vi "test Scripted Hardware Configuration.vi"(8 "error in (no error)":errorcluster, 11 "TestCase in":refnum<class "Hardware Configuration.lvclass">) -> (0 "error out":errorcluster, 3 "TestCase out":refnum<class "Hardware Configuration.lvclass">)   [LabVIEW 2020, in "Hardware Configuration.lvclass"]
uses:
  Hardware Configuration.lvclass
  <vilib>/addons/_JKI Toolkits/VI Tester/TestCase.llb/TestCase.lvclass
  niveristand-custom-device-testing-tools/Source/VeriStandTestUtilities/VeriStandTestUtilities.lvlib
  Scripting/Ballard/Ballard ARINC 429 Scripting.lvlib
  Hardware Configuration/Ballard ARINC 429 Hardware Configuration.lvlib
  C:/Program Files (x86)/National Instruments/LabVIEW 2020/vi.lib/addons/_JKI Toolkits/VI Tester/TestCase.llb/TestCase.lvclass
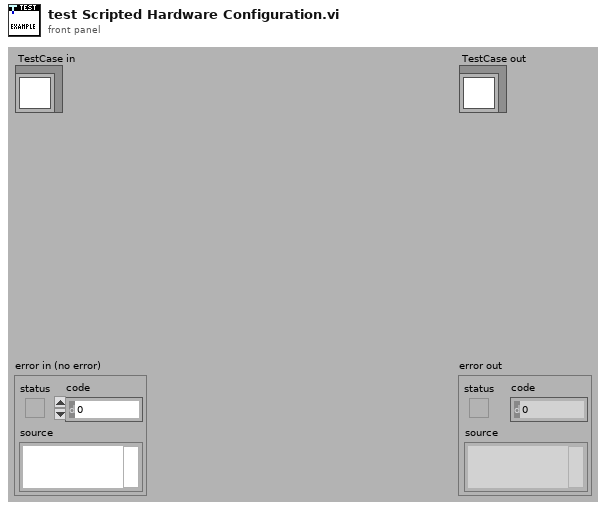
[diagram p1: front panel]
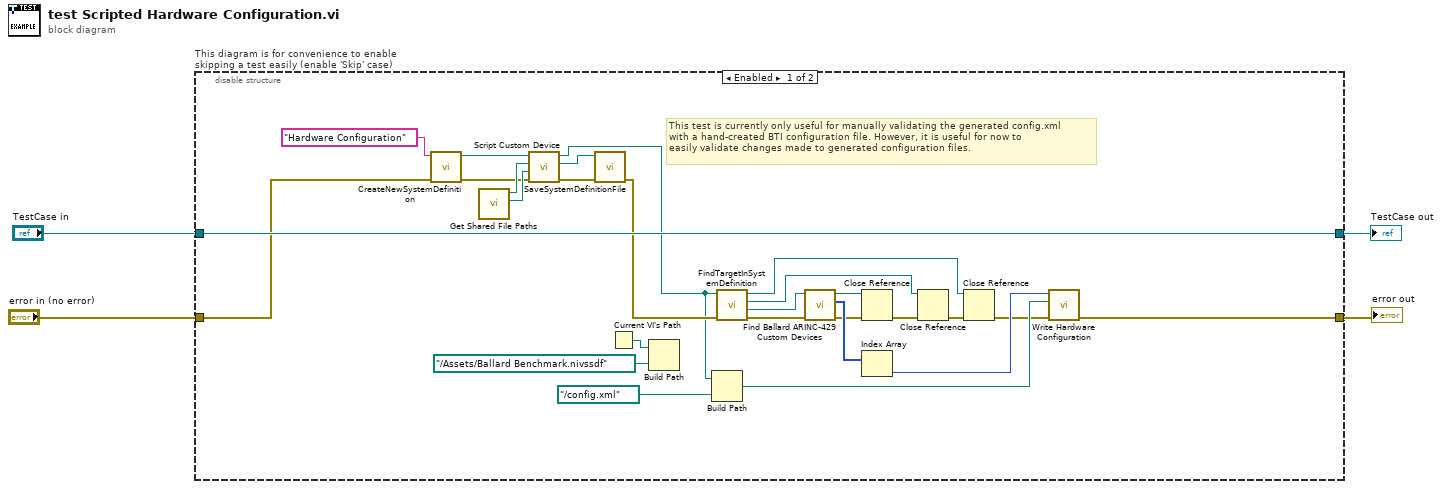
[diagram p0: block diagram]
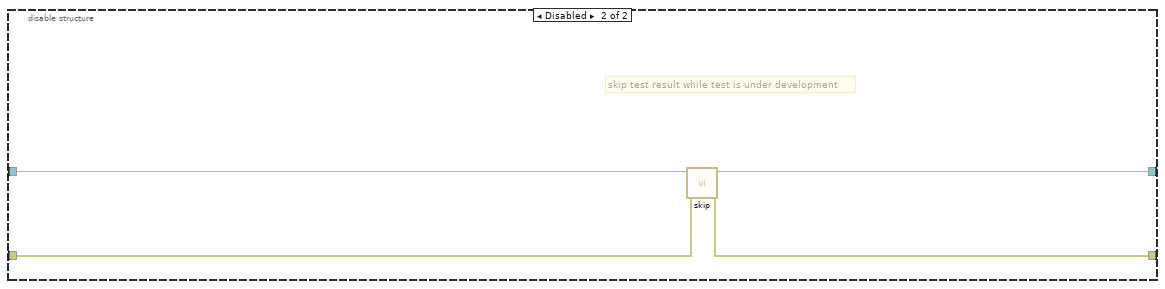
[diagram p2: hidden frame]
diagram:
  n1 = disable-structure "This diagram is for convenience to enable skipping a test easily (enable 'Skip' case)" shown="Enabled" {
    disable-tunnel: "TestCase in" -> [w31 w35]
    disable-tunnel: [w31 w33] -> w1
    disable-tunnel: [w17 w34] -> w3
    disable-tunnel: "error in (no error)" -> [w7 w32]
    frame Enabled {
      # "This test is currently only useful for manually validating the generated config.xml\nwith a hand-created BTI configuration file. However, it is useful for now to\neasily validate changes made to generated configuration files."
      n2 = call "CreateNewSystemDefinition.vi"("error in"=w7, "System Definition Name"="Hardware Configuration" ("Channel")) -> ("error out"=w10:errorcluster, "System Definition Path"=w12:path)  [unwired: 8 in]
      n3 = call "Get Shared File Paths.vi"() -> ("Hardware File"=w14:path, "Parameters File"=w13:path)  [unwired: 10 in]
      n4 = call "Script Custom Device.vi"("error in"=w10, "Hardware Configuration File Path"=w14, "Parameters Configuration File Path"=w13, "System Definition File Path In"=w12) -> ("error out"=w9:errorcluster, "System Definition Reference"=w11:refnum<k24>, "System Definition File Path Out"=w5:path)  [unwired: 4 in, 1 out]
      n5 = call "SaveSystemDefinitionFile.vi"("error in (no error)"=w9, "System Definition Reference in"=w11) -> ("error out"=w6:errorcluster)  [unwired: 8 in, 1 out]
      n6 = Current VI's Path() -> (path=w30:path)
      n7 = Build Path(base path=w30, name or relative path=path "../Assets/Ballard Benchmark.nivssdf") -> ()  [unwired: 1 out]
      n8 = Build Path(base path=w5, name or relative path=path "../config.xml") -> (appended path=w19:path)
      n9 = call "FindTargetInSystemDefinition.vi"("error in"=w6, "system definition path"=w5) -> ("error out"=w16:errorcluster, "Target"=w28:refnum<k24>, "Root"=w24:refnum<k24>, "System Definition"=w23:refnum<k24>)  [unwired: 6 in]
      n10 = call "Find Ballard ARINC-429 Custom Devices.vi"("error in"=w16, "target in"=w28) -> ("error out"=w15:errorcluster, "Ballard ARINC 429 custom devices"=w22:u64[], "target out"=w25:refnum<k24>)  [unwired: 7 in]
      n11 = Close Reference(reference=w25, error in (no error)=w15) -> (error out=w27:errorcluster)
      n12 = Index Array(array=w22) -> (element=w21:u64)  [unwired: 1 in]
      n13 = Close Reference(reference=w24, error in (no error)=w27) -> (error out=w26:errorcluster)
      n14 = Close Reference(reference=w23, error in (no error)=w26) -> (error out=w18:errorcluster)
      n15 = call "Write Hardware Configuration.vi"("error in"=w18, "path"=w19, "custom device"=w21) -> ("error out"=w17:errorcluster)  [unwired: 7 in, 1 out]
    }
    frame Disabled {
      # "skip test result while test is under development"
      n16 = call <vilib>:"skip.vi"("error in (no error)"=w32, "TestCase in"=w35) -> ("error out"=w34:errorcluster, "TestCase out"=w33:refnum<class "Hardware Configuration.lvclass">)  [unwired: 8 in]
    }
  }
  "error out" <- w3
  "TestCase out" <- w1
